vi "sub_generate-ray-casting-grid-map.vi"() -> ()   [LabVIEW 2019]
uses:
  Ctrl/cmd_common.ctl
  <vilib>/Analysis/Matrix/Numeric/Conversions/Array To Matrix - RA2.vi
  <vilib>/Analysis/Matrix/NI_Matrix.lvlib
panel:
  out "숫자형":i32
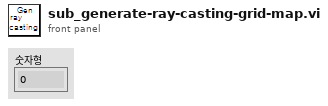
[diagram p1: front panel]
types:
  T1 = typedef "cmd_common.ctl" = enum16{"read", "write"}
  T2 = typedef "NI_Matrix.lvlib/RealMatrix.ctl" = dbl[][]
  T3 = cluster{"xy_resolution":dbl, "EXTEND_AREA":dbl, "MAX_RANGE":dbl, "NP":u32, "NTh":u32, "Q":T2, "R":T2, "Q_sim":T2, "R_sim":T2, "rf_id":cluster{"x":dbl, "y":dbl}[]}
  T4 = cluster{"ox":T2, "oy":T2, "occupancy map":T2, "x_true":T2, "u":T2, "z":T2, "PEst":T2, "min x":dbl, "min y":dbl, "max x":dbl, "max y":dbl, "yw":i32, "xw":i32, "center x":dbl, "center y":dbl}
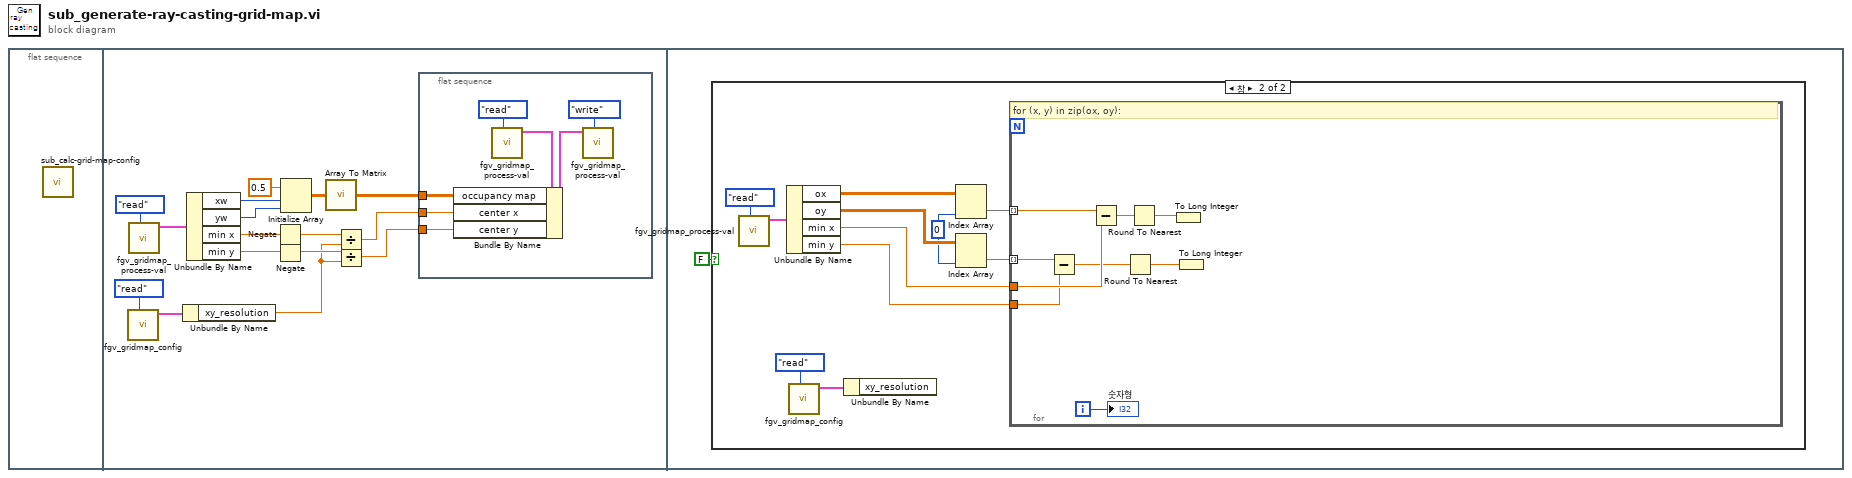
[diagram p0: block diagram]
diagram:
  n1 = flat-sequence {
    frame #0 {
      n2 = call "sub_calc-grid-map-config.vi"() -> ()  [unwired: 12 in]
    }
    frame #1 {
      n3 = call "fgv_gridmap_config.vi"("cmd"=cmd_common."read") -> ("pf-val out"=w5:T3)  [unwired: 10 in]
      n4 = call "fgv_gridmap_process-val.vi"("cmd"=cmd_common."read") -> ("p-val  2"=w15:T4)  [unwired: 10 in]
      n5 = Unbundle By Name(w5) -> ("xy_resolution"=w4:dbl)
      n6 = Unbundle By Name(w15) -> ("xw"=w14:i32, "yw"=w12:i32, "min x"=w10:dbl, "min y"=w9:dbl)
      n7 = Negate(x=w10) -> (-x=w8:dbl)
      n8 = Negate(x=w9) -> (-x=w7:dbl)
      n9 = Initialize Array(0.5 ("원소"), w14, w12) -> (w11:dbl[][])
      n10 = call-poly <vilib>:"Array To Matrix.vi"("Real 2D Array"=w11) -> ("Real Matrix"=w3:T2)
      n11 = Divide(x=w8, y=w4) -> (x/y=w2:dbl)
      n12 = Divide(x=w7, y=w4) -> (x/y=w1:dbl)
      n13 = flat-sequence {
        tunnel: w3 -> [w19]
        tunnel: w2 -> [w18]
        tunnel: w1 -> [w17]
        frame #0 {
          n14 = call "fgv_gridmap_process-val.vi"("cmd"=cmd_common."read") -> ("p-val  2"=w23:T4)  [unwired: 10 in]
          n15 = Bundle By Name(cluster=w23, "occupancy map"=w19, "center x"=w18, "center y"=w17) -> (w21:T4)
          n16 = call "fgv_gridmap_process-val.vi"("cmd"=cmd_common."write", "p-val"=w21) -> ()  [unwired: 9 in, 1 out]
        }
      }
    }
    frame #2 {
      n17 = case shown="참" FALSE {
        frame False {
        }
        frame True {
          w29 = 0 ("비활성화된 인덱스 (열)")
          n18 = call "fgv_gridmap_process-val.vi"("cmd"=cmd_common."read") -> ("p-val  2"=w35:T4)  [unwired: 10 in]
          n19 = Unbundle By Name(w35) -> ("ox"=w33:T2, "oy"=w32:T2, "min x"=w26:dbl, "min y"=w25:dbl)
          n20 = call "fgv_gridmap_config.vi"("cmd"=cmd_common."read") -> ("pf-val out"=w28:T3)  [unwired: 10 in]
          n21 = Unbundle By Name(w28) -> ()  [unwired: 1 out]
          n22 = Index Array(array=w33, index (col)=w29) -> (element=w31:dbl[])  [unwired: 1 in]
          n23 = Index Array(array=w32, index (col)=w29) -> (element=w30:dbl[])  [unwired: 1 in]
          n24 = for {
            tunnel: w31 -> [w43] mode=indexing
            tunnel: w30 -> [w41] mode=indexing
            tunnel: w26 -> [w42]
            tunnel: w25 -> [w40]
            i -> [w44]
            # "for (x, y) in zip(ox, oy):"
            n25 = Subtract(x=w41, y=w40) -> (x-y=w38:dbl)
            n26 = Subtract(x=w43, y=w42) -> (x-y=w39:dbl)
            n27 = Round To Nearest(number=w38) -> (nearest integer value=w36:dbl)
            n28 = Round To Nearest(number=w39) -> (nearest integer value=w37:dbl)
            n29 = To Long Integer(number=w37) -> ()  [unwired: 1 out]
            n30 = To Long Integer(number=w36) -> ()  [unwired: 1 out]
            "숫자형" <- w44
          }
        }
      }
    }
  }
